vi "initializeQueue.vi"(8 "error in (no error)":errorcluster, 11 "TCPCommunicator in":refnum<class "TCPCommunicator.lvclass">) -> (0 "error out":errorcluster, 3 "TCPCommunicator out":refnum<class "TCPCommunicator.lvclass">)   [LabVIEW 2016, in "TCPCommunicator.lvclass"]
uses:
  TCPCommunicator.lvclass
  TCPCommunicator.lvclass/TCPCommunicator.ctl
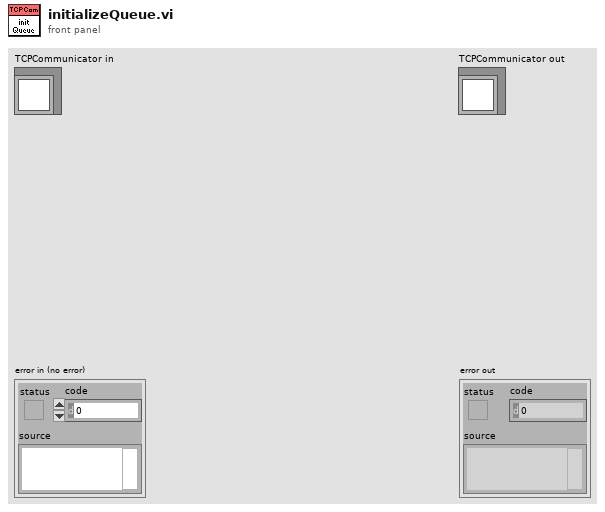
[diagram p1: front panel]
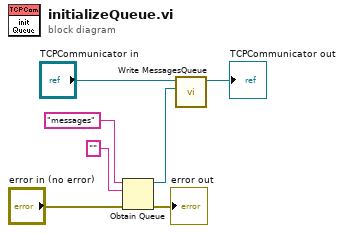
[diagram p0: block diagram]
diagram:
  n1 = Obtain Queue(name (unnamed)="messages", element data type="" ("name (unnamed)"), error in (no error)="error in (no error)") -> (queue out=w3:refnum<queue>, error out=→"error out":errorcluster)  [unwired: 2 in, 1 out]
  n2 = call "Write MessagesQueue.vi"("MessagesQueue"=w3, "TCPCommunicator in"="TCPCommunicator in") -> ("TCPCommunicator out"=→"TCPCommunicator out":refnum<class "TCPCommunicator.lvclass">)  [unwired: 8 in, 1 out]
